vi "GUIUpdater.vi"(0 "value":i8, 1 "Color":u32(colorbox), 2 "line":i8, 3 "MCListbox Refnum":refnum<vi>) -> ()   [LabVIEW 2009]
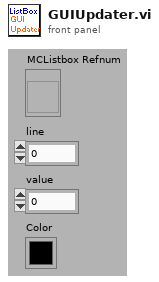
[diagram p1: front panel]
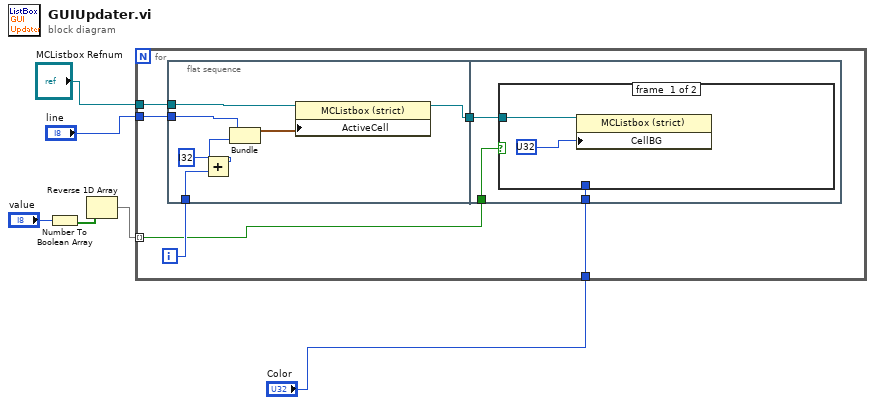
[diagram p0: block diagram]
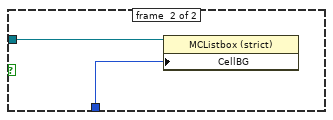
[diagram p2: hidden frame]
diagram:
  n1 = Number To Boolean Array(number="value") -> (Boolean array=w3:bool[])
  n2 = Reverse 1D Array(array=w3) -> (reversed array=w2:bool[])
  n3 = for {
    tunnel: w2 -> [w10] mode=indexing
    tunnel: "line" -> [w12]
    tunnel: "MCListbox Refnum" -> [w9]
    tunnel: "Color" -> [w7]
    i -> [w11]
    n4 = flat-sequence {
      tunnel: w12 -> [w14]
      tunnel: w11 -> [w18]
      tunnel: w9 -> [w15]
      tunnel: [w13] -> w8
      tunnel: w10 -> [w22]
      tunnel: w8 -> [w21]
      tunnel: w7 -> [w20]
      frame #0 {
        n5 = Add(x=i32 ?, y=w18) -> (x+y=w19:i32)
        n6 = Bundle("line"=w14, w19) -> (w16:cluster{"line":i8, i32})  [unwired: 1 in]
        n7 = property on="Property Node" class="MCListbox (strict)"(reference=w15, "ActiveCell"=w16) -> (reference out=w13:refnum<vi>)  [unwired: 1 in, 1 out]
      }
      frame #1 {
        n8 = case shown="True" w22 {
          tunnel: w21 -> [w23 w26]
          tunnel: w20 -> [_ w25]
          frame #0 {
            n9 = property on="Property Node" class="MCListbox (strict)"(reference=w23, "CellBG"=u32 ? ("Cell Background Color")) -> ()  [unwired: 1 in, 2 out]
          }
          frame #1 {
            n10 = property on="Property Node" class="MCListbox (strict)"(reference=w26, "CellBG"=w25) -> ()  [unwired: 1 in, 2 out]
          }
        }
      }
    }
  }
